vi "粘贴.vi"(8 "error in (no error)":errorcluster caption="错误输入（无错误）", 11 "程序响应 输入":refnum<class "程序响应.lvclass">) -> (0 "error out":errorcluster caption="错误输出", 3 "程序响应 输出":refnum<class "程序响应.lvclass">)   [LabVIEW 2020, in "程序响应.lvlib" / "程序响应.lvclass"]
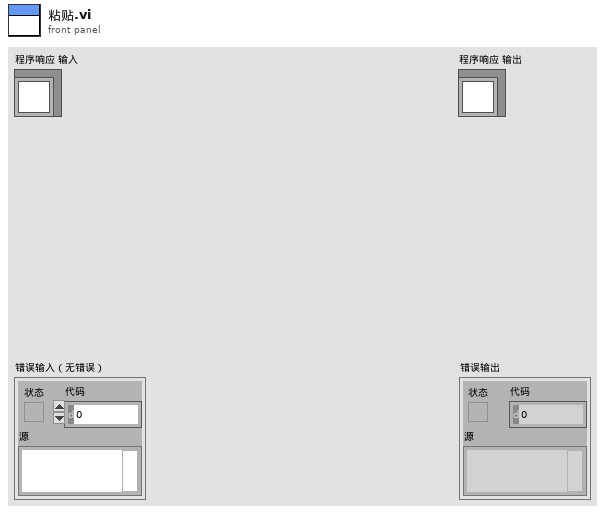
[diagram p1: front panel]
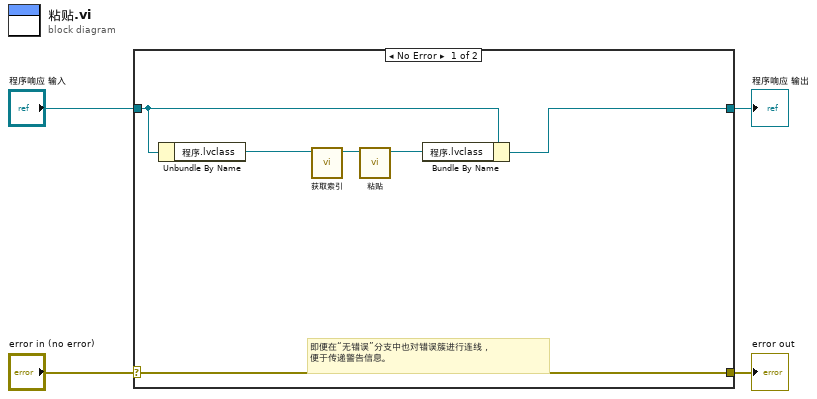
[diagram p0: block diagram]
diagram:
  n1 = case shown="No Error" "error in (no error)" {
    selector: "error in (no error)" -> [w10 w12]
    tunnel: [w10 w12] -> w3
    tunnel: [w7 w11] -> w1
    tunnel: "程序响应 输入" -> [w8 w11]
    frame No Error {
      # "即便在“无错误”分支中也对错误簇进行连线，\n便于传递警告信息。"
      n2 = Unbundle By Name(w8) -> ("程序.lvclass"=w5:refnum<class "程序.lvclass">)
      n3 = call-dynamic "获取索引.vi"("程序 输入"=w5) -> ("程序 输出"=w6:refnum<class "程序.lvclass">)  [unwired: 9 in, 1 out]
      n4 = call-dynamic "粘贴.vi"("程序 输入"=w6) -> ("程序 输出"=w9:refnum<class "程序.lvclass">)  [unwired: 9 in, 1 out]
      n5 = Bundle By Name(cluster=w8, "程序.lvclass"=w9) -> (w7:refnum<class "程序响应.lvclass">)
    }
    frame Error {
    }
  }
  "error out" <- w3
  "程序响应 输出" <- w1
